vi "Test Zip and Unzip.vi"() -> ()   [LabVIEW 2019]
uses:
  <vilib>/addons/_JKI Toolkits/Caraya/classes/Assert/Assert True.vi
  source/Command-Line Zip.lvlib
  <vilib>/addons/_JKI Toolkits/Caraya/classes/Test/Test.lvclass
  <vilib>/addons/_JKI Toolkits/Caraya/classes/Assert/Assert.lvclass
panel:
  out "temp folder location":path
  out "success zip/unzip single file?":bool
  in  "Delete Temp Folder on Success?":bool
  in  "error in":errorcluster
  out "success zip/unzip folder?":bool
  out "error out":errorcluster
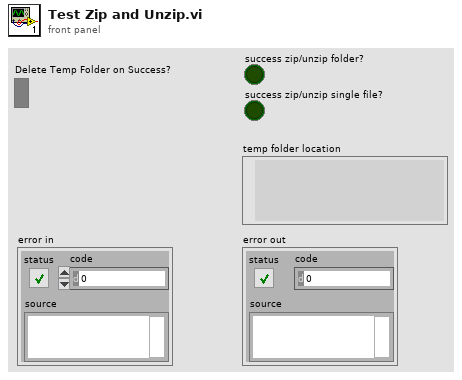
[diagram p1: front panel]
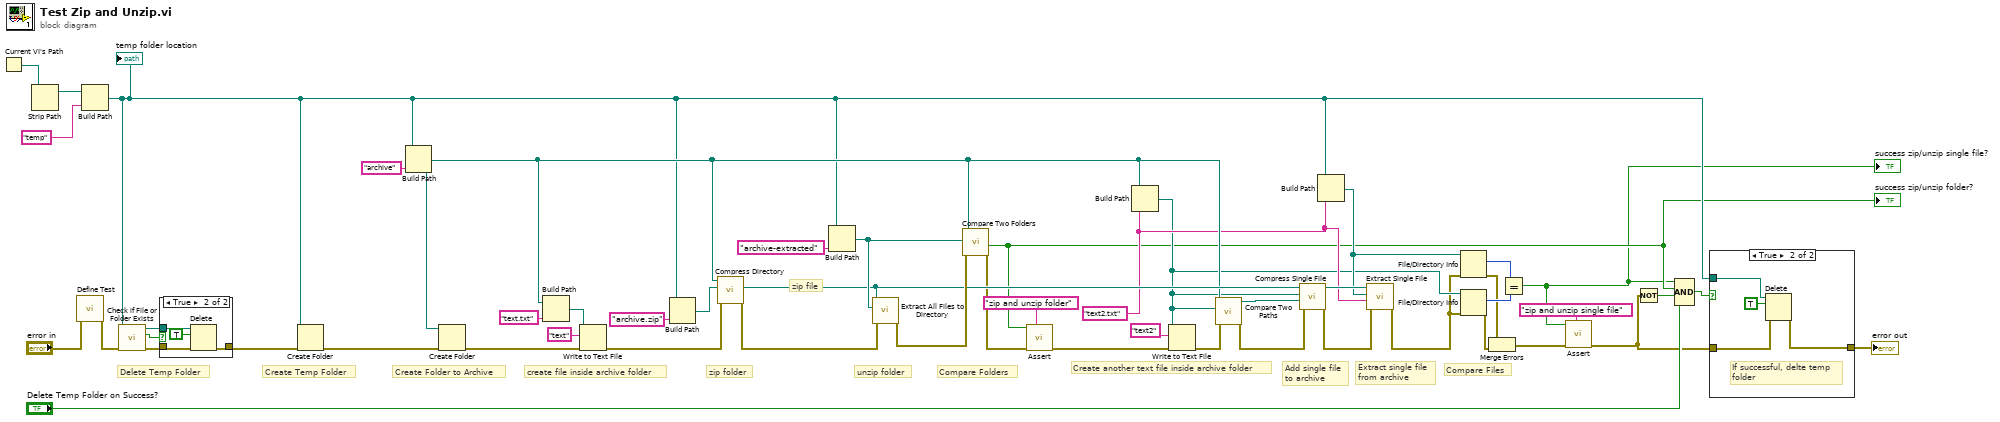
[diagram p0: block diagram]
diagram:
  w20 = "text2.txt" ("name or relative path")
  # "Extract single file from archive"
  # "Add single file to archive"
  # "Create another text file inside archive folder"
  # "Compare Files"
  # "zip file"
  # "unzip folder"
  # "Compare Folders"
  # "zip folder"
  # "create file inside archive folder"
  # "Create Folder to Archive"
  # "Create Temp Folder"
  # "Delete Temp Folder"
  n1 = Current VI's Path() -> (path=w51:path)
  n2 = Strip Path(path=w51) -> (stripped path=w50:path)  [unwired: 1 out]
  n3 = call <vilib>:"Define Test.vi"("error in (no error)"="error in") -> ("error out"=w9:errorcluster)  [unwired: 10 in]
  n4 = Build Path(base path=w50, name or relative path="temp") -> (appended path=w21:path)
  "temp folder location" <- w21
  n5 = call <vilib>:"Check if File or Folder Exists.vi"("error in (no error)"=w9, "path"=w21) -> ("error out"=w34:errorcluster, "file or folder exists?"=w31:bool, "dup path"=w32:path)  [unwired: 7 in]
  n6 = case shown="True" w31 {
    tunnel: w34 -> [w52 w55]
    tunnel: [w52 w54] -> w33
    tunnel: w32 -> [_ w53]
    frame False {
    }
    frame True {
      n7 = Delete(path (use dialog)=w53, entire hierarchy (F)=TRUE, error in=w55) -> (error out=w54:errorcluster)  [unwired: 2 in, 2 out]
    }
  }
  n8 = Create Folder(path (use dialog)=w21, error in=w33) -> (error out=w48:errorcluster)  [unwired: 1 in, 2 out]
  n9 = Build Path(base path=w21, name or relative path="archive") -> (appended path=w25:path)
  n10 = Create Folder(path (use dialog)=w25, error in=w48) -> (error out=w46:errorcluster)  [unwired: 1 in, 2 out]
  n11 = Build Path(base path=w25, name or relative path="text.txt") -> (appended path=w44:path)
  n12 = Write to Text File(file (use dialog)=w44, text="text", error in=w46) -> (error out=w42:errorcluster)  [unwired: 1 in, 2 out]
  n13 = Build Path(base path=w21, name or relative path="archive.zip") -> (appended path=w39:path)
  n14 = call "Compress Directory.vi"("error in (no error)"=w42, "archive name (root directory with .zip ending)"=w39, "root directory (file dialog)"=w25) -> ("error out"=w41:errorcluster, "archive name out"=w27:path)  [unwired: 6 in, 1 out]
  n15 = Build Path(base path=w21, name or relative path="archive-extracted") -> (appended path=w30:path)
  n16 = call "Extract All Files to Directory.vi"("error in (no error)"=w41, "Extract to Dir"=w30, "Zip File Path"=w27) -> ("error out"=w29:errorcluster)  [unwired: 8 in]
  n17 = call "Compare Two Folders.vi"("error in (no error)"=w29, "appended path 2"=w30, "appended path"=w25) -> ("error out"=w7:errorcluster, "Contents are the same?"=w8:bool)  [unwired: 7 in]
  "success zip/unzip folder?" <- w8
  n18 = call-poly <vilib>:"Assert.vi"("Label"="zip and unzip folder", "error in (no error)"=w7, "True?"=w8) -> ("error out"=w6:errorcluster)  [unwired: 8 in]
  n19 = Build Path(base path=w25, name or relative path=w20) -> (appended path=w17:path)
  n20 = Write to Text File(file (use dialog)=w17, text="text2", error in=w6) -> (error out=w24:errorcluster)  [unwired: 1 in, 2 out]
  n21 = call <vilib>:"Compare Two Paths.vi"("error in (no error)"=w24, "Path 2"=w17, "Path 1"=w25) -> ("error out"=w23:errorcluster, "Relative Path from 1 to 2"=w11:path)  [unwired: 5 in, 2 out]
  n22 = call "Compress Single File.vi"("error in (no error)"=w23, "Internal Name"=w11, "Source File Path"=w17, "Zip File Path"=w27) -> ("error out"=w19:errorcluster, "dup Zip File Path"=w22:path)  [unwired: 5 in, 1 out]
  n23 = Build Path(base path=w21, name or relative path=w20) -> (appended path=w18:path)
  n24 = call "Extract Single File.vi"("error in (no error)"=w19, "name or relative path (\"\": use output file name)"=w20, "File output Path (extract to temp file)"=w18, "Zip File Path"=w22) -> ("error out"=w16:errorcluster)  [unwired: 4 in, 3 out]
  n25 = File/Directory Info(path=w18, error in=w16) -> (size=w15:i64, error out=w13:errorcluster)  [unwired: 5 out]
  n26 = File/Directory Info(path=w17, error in=w16) -> (size=w14:i64, error out=w12:errorcluster)  [unwired: 5 out]
  n27 = Merge Errors(w13, w12) -> (w4:errorcluster)
  n28 = Equal?(x=w15, y=w14) -> (x = y?=w2:bool)
  "success zip/unzip single file?" <- w2
  n29 = call-poly <vilib>:"Assert.vi"("Label"="zip and unzip single file", "error in (no error)"=w4, "True?"=w2) -> ("error out"=w3:errorcluster)  [unwired: 8 in]
  n30 = Not(x=w3) -> (.not. x?=w35:bool)
  n31 = Compound Arithmetic op=AND(w2, w8, w35, "Delete Temp Folder on Success?") -> (w36:bool)
  n32 = case shown="True" w36 {
    tunnel: [w57 w58] -> w37
    tunnel: w3 -> [w57 w59]
    tunnel: w21 -> [_ w60]
    frame False {
    }
    frame True {
      # "If successful, delte temp folder"
      n33 = Delete(path (use dialog)=w60, entire hierarchy (F)=TRUE, error in=w59) -> (error out=w58:errorcluster)  [unwired: 2 in, 2 out]
    }
  }
  "error out" <- w37
